vi "sv_SDOF Shock Response (Norm).vi"(6 "model":i32(ring) items=["Absolute acceleration", "Relative displacement"], 8 "error in (no error)":errorcluster, 9 "critical damping factor":dbl=0.05 format="%.2f", 10 "fn [Hz]":dbl=100.0 format="%.2f", 11 "scaled signal [EU]":waveform(dbl)) -> (0 "error out":errorcluster, 3 "SDOF shock response":waveform(dbl))   [LabVIEW 2017, in "SoundVib_Transient.lvlib"]
uses:
  <vilib>/addons/Sound and Vibration/svt_Transients/SoundVib_Transient.lvlib
  <vilib>/Analysis/3filter.llb/IIR Filter (DBL).vi
  <vilib>/Analysis/NI_AALBase.lvlib
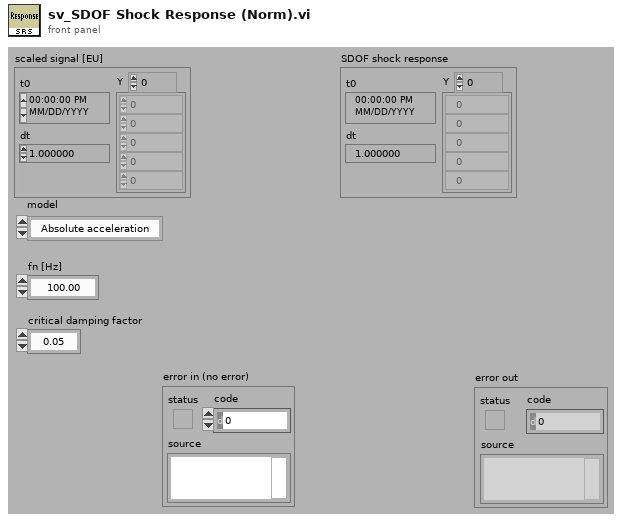
[diagram p1: front panel]
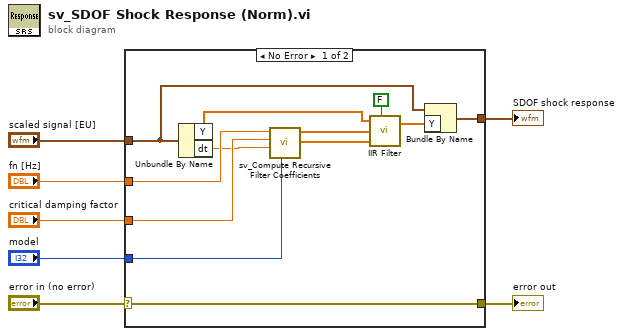
[diagram p0: block diagram]
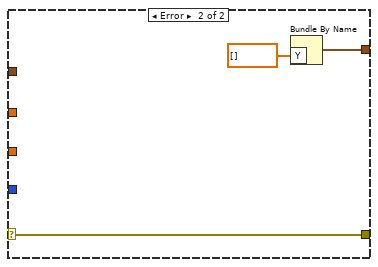
[diagram p2: hidden frame]
diagram:
  n1 = case shown="No Error" "error in (no error)" {
    selector: "error in (no error)" -> [w14 w22]
    tunnel: "scaled signal [EU]" -> [w18 _]
    tunnel: "fn [Hz]" -> [w13 _]
    tunnel: "critical damping factor" -> [w12 _]
    tunnel: [w15 w21] -> w4
    tunnel: "model" -> [w10 _]
    tunnel: [w14 w22] -> w1
    frame No Error {
      n2 = Unbundle By Name(w18) -> ("Y"=w17:dbl[], "dt"=w11:dbl)
      n3 = call <vilib>:"sv_Compute Recursive Filter Coefficients.vi"("model"=w10, "dt [s]"=w11, "critical damping factor"=w12, "fn [Hz]"=w13) -> ("forward coefficients"=w8:dbl[], "reverse coefficients"=w9:dbl[])  [unwired: 6 in]
      n4 = call-poly <vilib>:"IIR Filter.vi"("init/cont (init:F)"=FALSE, "Forward Coefficients"=w8, "Reverse Coefficients"=w9, "X"=w17) -> ("Filtered X"=w16:dbl[])  [unwired: 1 out]
      n5 = Bundle By Name(cluster=w18, "Y"=w16) -> (w15:waveform(dbl))
    }
    frame Error {
      n6 = Bundle By Name("Y"=dbl[] []) -> (w21:waveform(dbl))  [unwired: 1 in]
    }
  }
  "SDOF shock response" <- w4
  "error out" <- w1
